vi "lab4.vi"() -> ()   [LabVIEW 2016]
panel:
  out "Area":dbl
  in  "A":dbl
  in  "C":dbl
  in  "B":dbl
  out "S":dbl
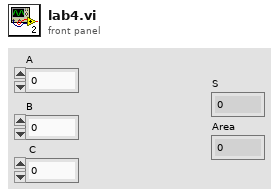
[diagram p1: front panel]
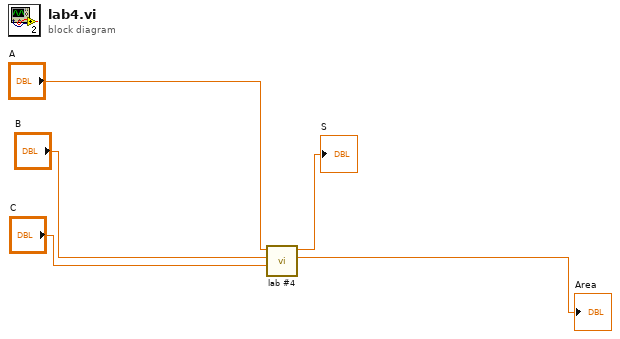
[diagram p0: block diagram]
diagram:
  n1 = call "lab #4.vi"("C"="C", "B"="B", "A"="A") -> ("Area"=→"Area":dbl, "S"=→"S":dbl)  [unwired: 7 in]
